vi "Data.vi"(11 "Panel Create Msg Strategy in":refnum<class "Panel Create Msg Strategy.lvclass">) -> (2 "Panel":refnum<class "Panel.lvclass">)   [LabVIEW 2021, in "Panel Create.lvlib" / "Panel Create Msg Strategy.lvclass"]
uses:
  Panel Create Msg Strategy.lvclass
  Panel Create Msg Strategy.lvclass/Panel Create Msg Strategy.ctl
  Panel/Panel.lvclass
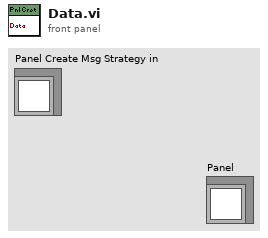
[diagram p1: front panel]
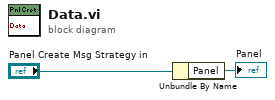
[diagram p0: block diagram]
diagram:
  n1 = Unbundle By Name("Panel Create Msg Strategy in") -> ("Panel"=→"Panel":refnum<class "Panel.lvclass">)
